vi "Generate Random Lorem Ipsum Error Message.vi"(1 "Dummy Error Message Length":T1=enum."Medium (Up to 1,000 characters)") -> (0 "Random Lorem Ipsum Error Message (dummy error message)":string)   [LabVIEW 2016, in "Simple Tester.lvclass"]
doc: "This VI generates dummy error message. The error messages are based on the Lorem Ipsum text, and are of random lengths."
uses:
  Simple Tester.lvclass
  Dummy Error Message Length (enum).ctl
panel:
  out "Dummy Error Message Length":i32
  out "End index":u32
  out "Input Lorem Ipsum text length":u32
  out "Start index (confirmed)":u32
  out "Start index (randomly chosen)":u32
  # "Development\nControls or indicators that are useful for development or testing, but which are not outputs of the VI."
  # "Input\nInputs to the VI"
  # "Output\nOutputs of the VI"
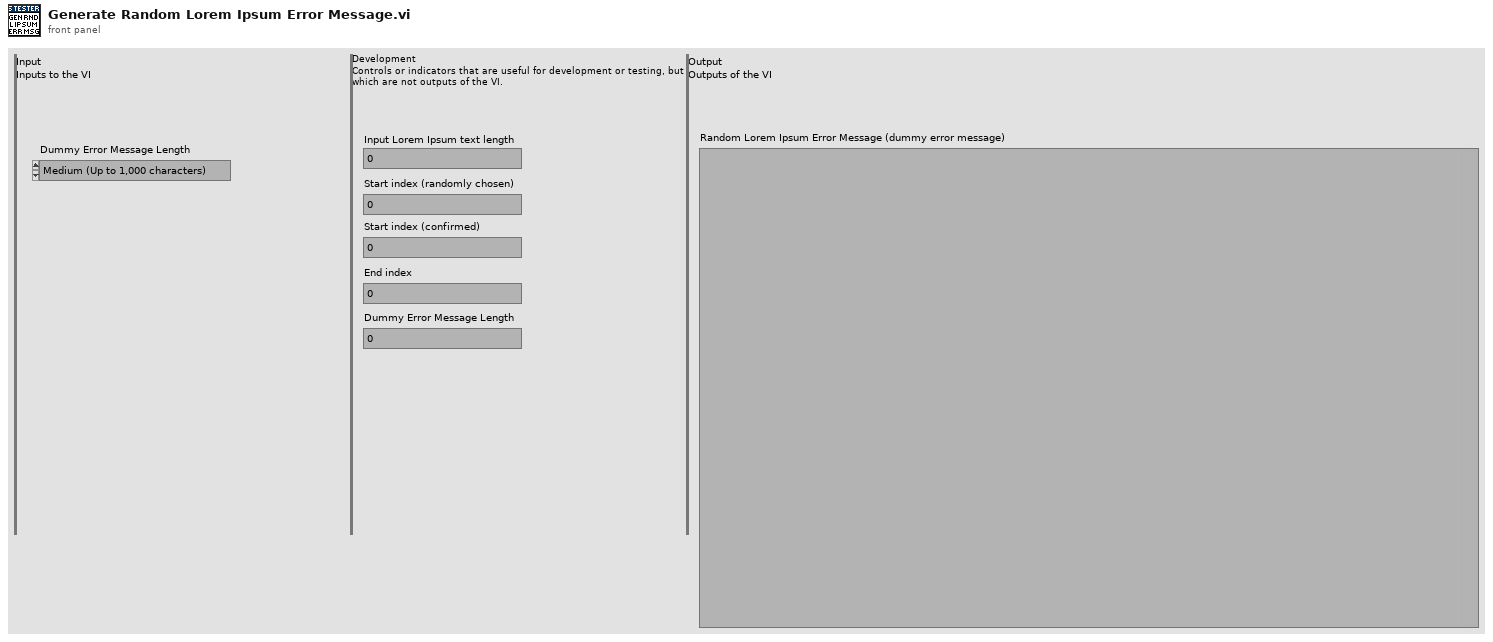
[diagram p1: front panel]
types:
  T1 = typedef "Simple Tester.lvclass/Dummy Error Message Length (enum).ctl" = enum16{"Short (Up to 100 characters)", "Medium (Up to 1,000 characters)", "Long (Up to 10,000 characters)"}
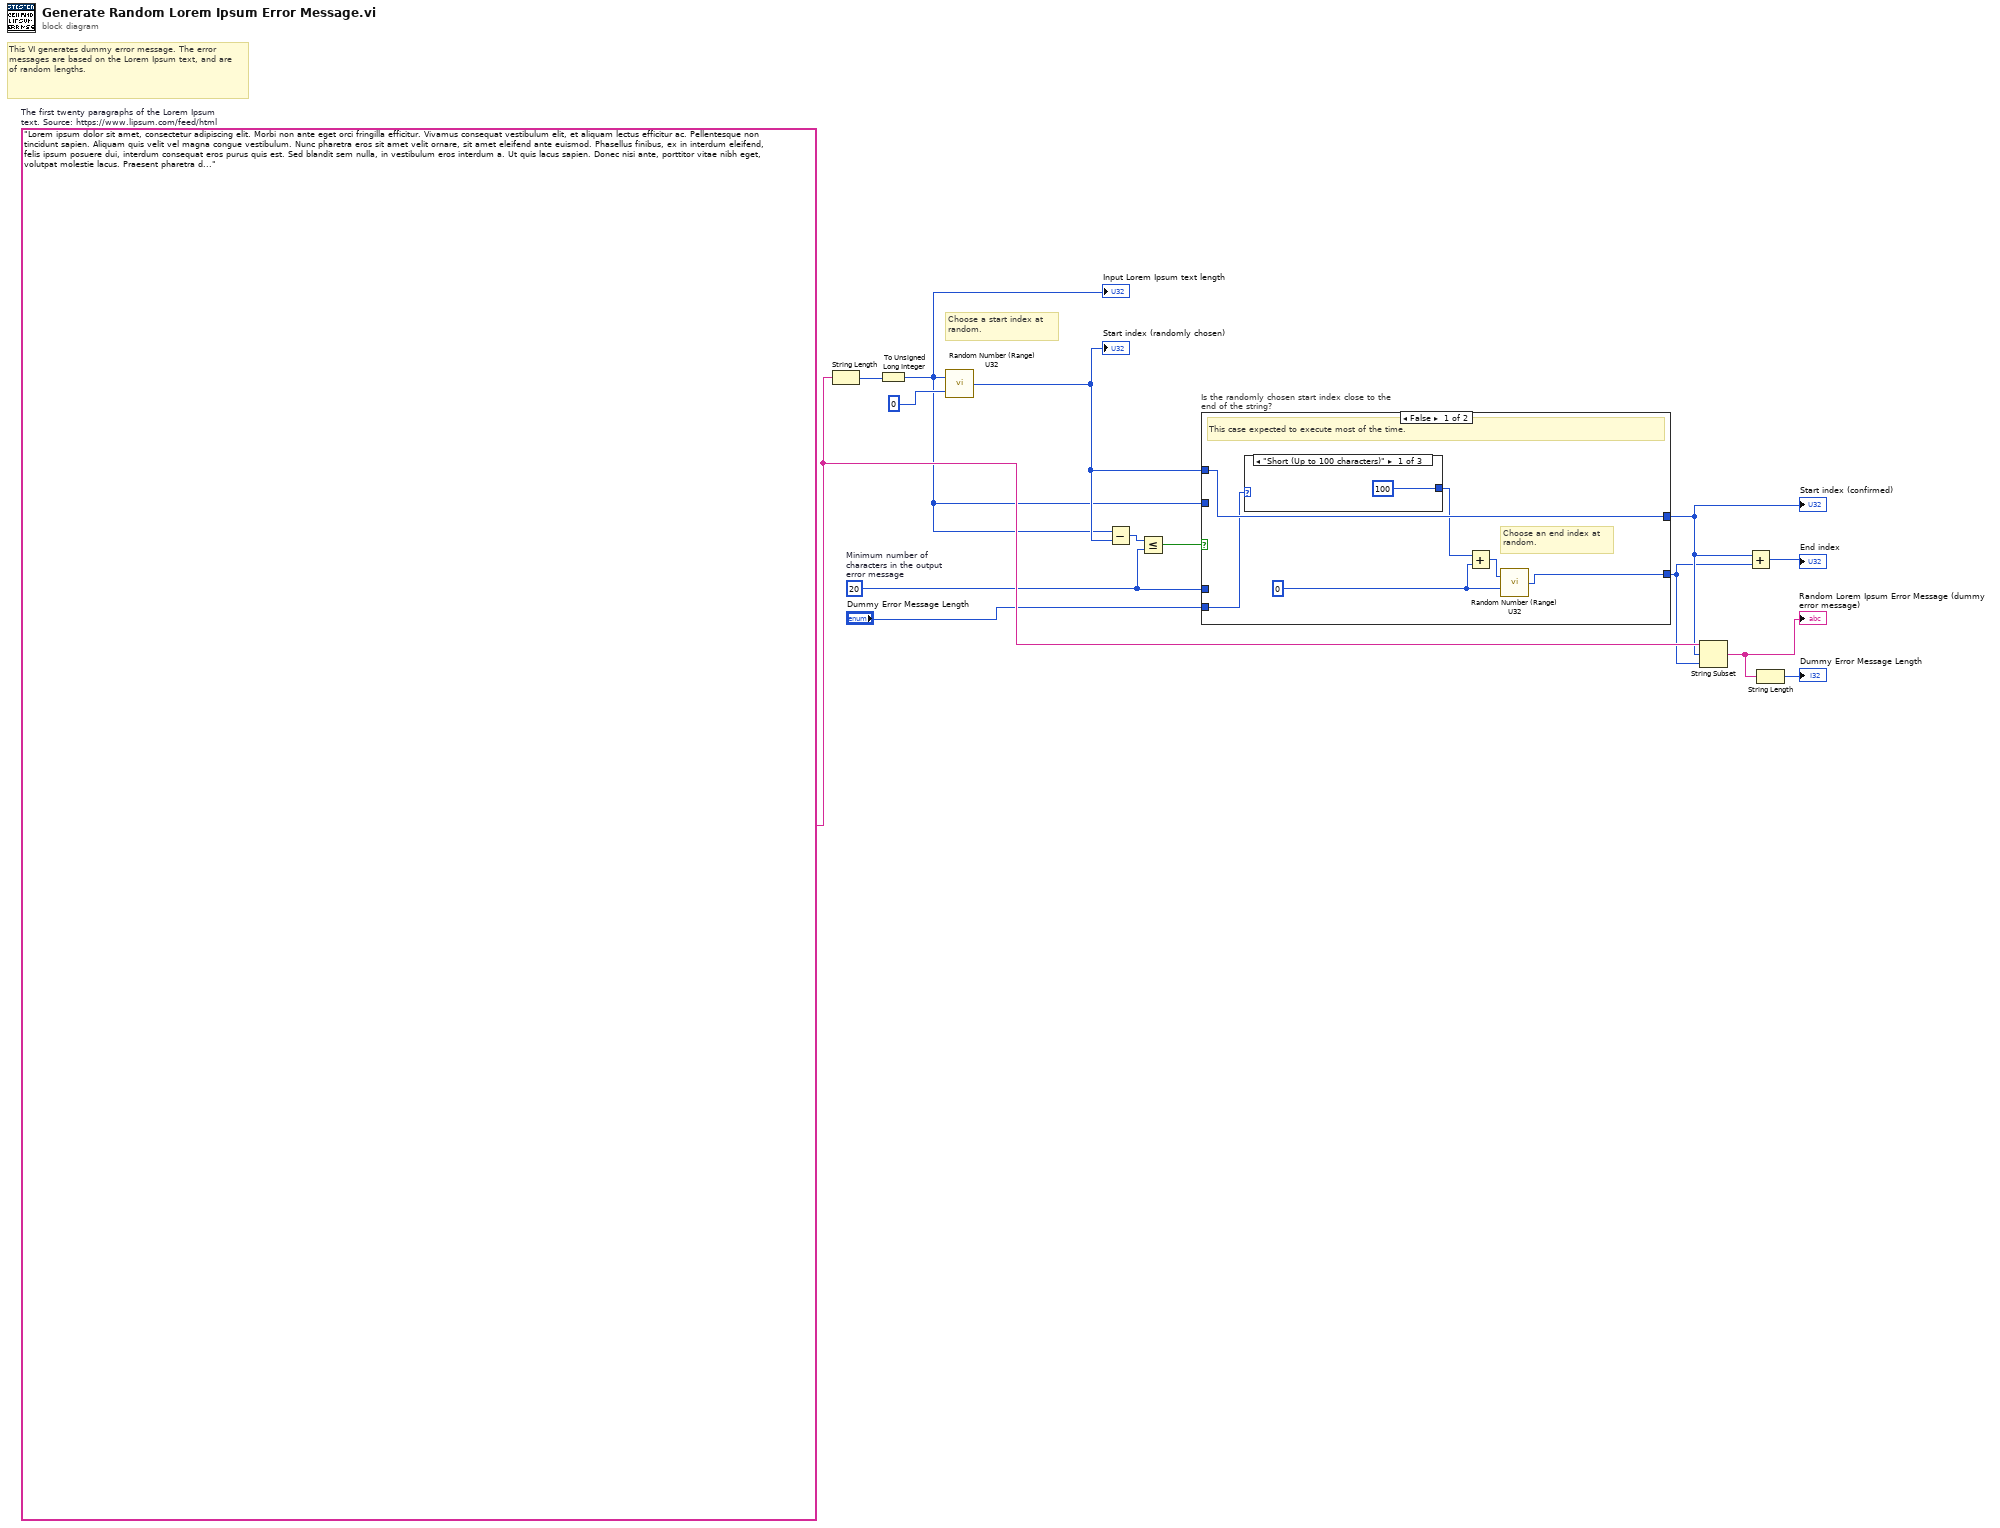
[diagram p0: block diagram]
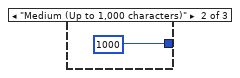
[diagram p2: hidden frame]
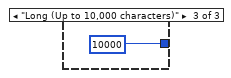
[diagram p3: hidden frame]
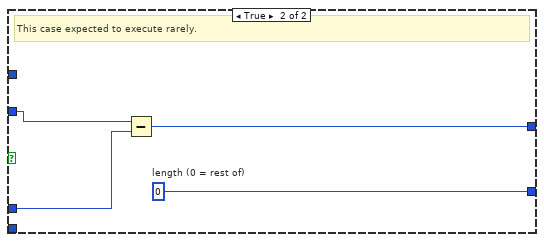
[diagram p4: hidden frame]
diagram:
  w10 = u32 20  # Minimum number of characters in the output error message
  w13 = "Lorem ipsum dolor sit amet, consectetur adipiscing elit. Morbi non ante eget orci fringilla efficitur. Vivamus consequat vestibulum elit, et aliquam lectus efficitur ac. Pellentesque non tincidunt sapien. Aliquam quis velit vel magna congue vestibulum. Nunc pharetra eros sit amet velit ornare, sit amet eleifend ante euismod. Phasellus finibus, ex in interdum eleifend, felis ipsum posuere dui, interdum consequat eros purus quis est. Sed blandit sem nulla, in vestibulum eros interdum a. Ut quis lacus sapien. Donec nisi ante, porttitor vitae nibh eget, volutpat molestie lacus. Praesent pharetra diam vitae dolor cursus, sed finibus tellus convallis. Nullam et sodales dui. Aliquam vehicula pellentesque odio, sed mattis leo gravida consectetur. Aliquam fermentum ex lacus, eget venenatis erat tincidunt vitae. Cras pharetra lacinia elit nec pulvinar.\n\nIn hac habitasse platea dictumst. Donec sit amet quam non justo pharetra lobortis id in justo. Suspendisse aliquet lectus venenatis aliquet scelerisque. Sed imperdiet dictum enim, nec maximus dui pretium condimentum. Aenean vel facilisis eros, et vestibulum mauris. Donec eget libero aliquet, suscipit augue eu, dapibus sapien. Phasellus nunc dui, suscipit sed dui vitae, sollicitudin lacinia turpis.\n\nMaecenas sit amet augue at orci aliquet accumsan a ut mi. Suspendisse ultrices tellus quis nibh pretium luctus. Curabitur sapien orci, pharetra at ligula sit amet, dapibus pulvinar augue. Nullam risus risus, sollicitudin in molestie sed, suscipit ut arcu. Suspendisse non suscipit quam. Quisque fringilla id ante a vehicula. Donec vel maximus ante. Vivamus ut hendrerit lectus. Nunc tincidunt vel nibh id tristique. Pellentesque aliquet libero rutrum tortor vulputate, quis euismod turpis blandit. Phasellus efficitur feugiat convallis. Aliquam lectus ipsum, sodales et velit vel, iaculis mollis est. Nulla quis varius elit. Duis massa elit, feugiat non massa non, interdum dignissim urna. Nunc at velit quis nisl mollis blandit nec sit amet nisi. Sed dignissim ex eu tincidunt ultricies.\n\nUt commodo tempus elit, ac tincidunt dui vehicula et. Suspendisse convallis ante sit amet felis semper ultrices. Donec ultricies bibendum lacus nec laoreet. Etiam ullamcorper felis tellus, in mattis felis pulvinar molestie. Aenean et velit a lacus gravida scelerisque nec ac odio. Aliquam erat volutpat. Nulla facilisi. Maecenas id augue mauris. Ut tempus leo et lectus ultrices elementum. Duis posuere, nisl eget elementum sagittis, justo leo mattis tellus, id aliquam ipsum leo in dui. Praesent ut nisi non ante lobortis gravida. Donec id sem orci.\n\nNam sed lectus sed orci maximus volutpat id et nisi. Vestibulum vulputate consectetur velit et dictum. Sed sit amet ex lacus. Orci varius natoque penatibus et magnis dis parturient montes, nascetur ridiculus mus. Donec consequat lorem sit amet tellus aliquam, at vehicula velit viverra. Sed ipsum turpis, volutpat ac justo eu, suscipit pharetra eros. Duis bibendum auctor orci sit amet eleifend. Vivamus turpis neque, fringilla vitae mattis ac, consequat vel turpis. Donec dapibus sapien eu mauris viverra, a interdum augue lobortis. Nullam vitae ultrices ex. Nulla in purus porttitor elit fringilla sagittis.\n\nQuisque fermentum massa quis lectus finibus faucibus. Nulla aliquet ac arcu in sagittis. Suspendisse nec massa ullamcorper, porta nulla quis, rhoncus enim. Sed ornare rhoncus nulla, sed fringilla ex tincidunt eget. Sed varius ipsum ligula, eu sollicitudin eros lobortis ut. Maecenas tristique nulla erat, sed faucibus erat rhoncus a. Nam elementum nisl quis est cursus, ac tempor mauris feugiat.\n\nDonec vitae maximus justo. Morbi sapien lorem, elementum at pellentesque sed, luctus eu quam. Ut congue efficitur eros id egestas. In ac nunc sed elit ultricies pellentesque. Donec et velit ac ante efficitur malesuada vel sed mi. Donec convallis, mi lacinia convallis tristique, nunc dolor elementum sapien, ac mollis magna sapien a felis. Vivamus at purus pellentesque mauris eleifend tincidunt ut at augue. Suspendisse tristique erat nec neque tristique finibus vel quis nunc. Cras posuere eros mauris, sed ultrices arcu auctor interdum. Quisque ac elit commodo, tempor urna eget, viverra ante. Vestibulum auctor elit sit amet leo blandit, mattis tempus tellus auctor. Donec mollis sem et urna aliquam, at consectetur mi bibendum. Vivamus pellentesque, ex id ullamcorper molestie, justo mauris hendrerit nunc, vitae pretium elit mi ac diam. Praesent efficitur ligula vitae ex ultrices, eget pulvinar purus posuere.\n\nSed efficitur mollis odio, vel semper lorem tempor id. Maecenas blandit arcu eu ante malesuada finibus. Curabitur ut nunc consequat, laoreet risus ac, rhoncus enim. Cras diam neque, consectetur vel faucibus et, pulvinar sed quam. Nam quis feugiat est, eu viverra velit. Maecenas consequat tortor urna, ut facilisis lectus ultrices et. Pellentesque dictum leo id ex tincidunt, sit amet bibendum arcu pretium. Cras maximus facilisis ornare. Integer efficitur augue quis magna tristique, sed scelerisque urna placerat. Etiam ornare neque lectus, eget gravida orci vestibulum nec.\n\nSuspendisse hendrerit congue lorem vel consectetur. Vivamus purus nulla, condimentum vel auctor ut, dignissim vel mi. Lorem ipsum dolor sit amet, consectetur adipiscing elit. Curabitur non gravida ex. Morbi sodales sem id justo eleifend pretium. Duis aliquam mi ut leo ornare porta. Phasellus vehicula tortor mi, a hendrerit elit ultrices vitae. Curabitur nec rutrum orci, non venenatis leo. Maecenas hendrerit orci eu tincidunt efficitur. Integer fringilla finibus iaculis.\n\nNulla facilisi. Proin id mi nec lectus varius aliquam. Nulla porta, velit in varius volutpat, libero massa interdum metus, sit amet mattis est lorem nec felis. Vestibulum ante ipsum primis in faucibus orci luctus et ultrices posuere cubilia curae; Integer aliquam malesuada justo, quis porta quam ultrices in. Nam nec interdum lorem. Praesent metus enim, eleifend a neque nec, aliquet imperdiet erat.\n\nPhasellus tortor justo, tincidunt vitae tempor nec, aliquam nec ipsum. Nulla gravida tortor vel metus efficitur, ut rutrum libero vestibulum. Suspendisse rutrum auctor massa rutrum ullamcorper. In hac habitasse platea dictumst. Integer feugiat vel dui et maximus. Morbi eu mauris eget lectus efficitur vestibulum nec quis libero. Etiam at lectus pellentesque, maximus nisl a, tristique odio. Vivamus pretium libero id justo vestibulum imperdiet.\n\nNulla eu tellus pharetra, egestas nibh ut, vehicula quam. Duis vitae odio non risus hendrerit viverra eget eget enim. Nam eleifend, felis eget vehicula varius, enim nunc facilisis neque, vitae tincidunt eros tortor eget erat. Sed ultrices sapien nibh, vitae maximus ex rutrum sit amet. Nullam in ipsum ut velit maximus mollis nec ultricies urna. Duis et egestas orci. Quisque non magna tortor. In imperdiet tortor diam, eget commodo nunc varius et. In hendrerit imperdiet tellus vitae mollis.\n\nUt euismod nulla id augue elementum, non tempor nibh vulputate. Mauris vulputate ut massa quis vulputate. Nullam tristique elit nisl, sed dignissim mi sollicitudin eu. Vivamus cursus neque mauris, vitae feugiat augue aliquam sit amet. Cras efficitur, nunc vitae tincidunt iaculis, ante orci fermentum leo, vel hendrerit leo est fermentum ligula. Nullam sed erat vitae justo dapibus mattis. Phasellus rutrum scelerisque risus. Nunc auctor sed arcu non venenatis. Ut lectus tellus, semper sit amet nunc vel, dapibus bibendum nunc. Sed interdum, nunc eget rhoncus lacinia, nunc orci ornare nibh, porttitor faucibus arcu elit ut sapien. Suspendisse potenti. Duis ligula augue, facilisis id tellus sed, malesuada tristique erat. Nam fermentum lorem diam, vitae bibendum mauris condimentum nec.\n\nNulla at velit massa. Etiam eu justo ut dui pretium sodales. Aliquam in justo ex. Integer lacinia nunc ut eros porta, quis venenatis felis mattis. Pellentesque elementum nunc lobortis, dictum sem non, bibendum ante. Nulla efficitur ultrices sapien, nec lacinia orci malesuada id. Nullam maximus arcu felis, ac rhoncus quam euismod a. Nam luctus, diam non pulvinar viverra, massa ante mollis massa, ac venenatis lorem odio nec nisi. Nam molestie gravida risus, eu pellentesque erat tincidunt laoreet. Orci varius natoque penatibus et magnis dis parturient montes, nascetur ridiculus mus. Maecenas consequat vestibulum nisl, et malesuada felis commodo ut. Aliquam tincidunt, tellus in egestas dignissim, eros elit sodales metus, vel porttitor odio orci id tortor. Nulla congue condimentum eleifend. Duis a purus elit. In pretium, nisl sit amet volutpat sagittis, mi orci malesuada odio, eget placerat enim purus in lorem. Maecenas molestie velit et lacus posuere, ac mattis massa posuere.\n\nPhasellus dignissim erat in mi semper vehicula. Sed mauris dolor, venenatis ut ullamcorper et, tempor at diam. In euismod vestibulum magna ut sodales. Sed imperdiet condimentum semper. Nunc vel erat at orci posuere semper. Cras sapien purus, auctor quis auctor id, ultrices ac magna. Etiam gravida nec urna eget maximus. Nulla convallis vestibulum nisi, a elementum tortor placerat ac. Nulla ornare aliquet vehicula. Cras ac est a quam pharetra venenatis in ut leo.\n\nNullam ac augue fermentum, commodo justo ac, molestie leo. Integer vitae sollicitudin leo, vel vehicula nisi. Morbi id nulla eu nulla scelerisque euismod. Cras posuere tellus ac risus consequat molestie. Vestibulum et rutrum ante. Quisque pharetra est a consequat ultrices. Maecenas ac molestie neque. Aenean facilisis mauris nec felis laoreet auctor. Vestibulum posuere finibus pellentesque. Mauris ultricies nec libero ac placerat. Ut congue arcu et tincidunt lacinia. Vestibulum sem mi, venenatis id erat ut, mattis fermentum neque.\n\nNunc ante ipsum, viverra eget tincidunt quis, elementum mollis eros. Sed euismod vehicula orci vitae lobortis. Curabitur aliquet, urna quis suscipit blandit, nibh mi malesuada dolor, pharetra feugiat augue lacus eget urna. Nam neque felis, tristique et sapien vel, sollicitudin posuere lectus. Vivamus eget finibus nunc, eu hendrerit mauris. Phasellus pulvinar turpis non auctor hendrerit. Fusce et mi tincidunt, aliquam nulla sit amet, ullamcorper metus. Nunc eget sem eu leo semper dictum. In consequat vestibulum velit interdum laoreet. Etiam interdum neque accumsan varius consequat. Nullam interdum, mi non tristique dictum, metus erat blandit tortor, at dignissim mi ligula et enim.\n\nProin ornare rutrum orci id bibendum. Sed consequat pharetra massa nec faucibus. Vestibulum id odio vel diam sagittis posuere. Nulla vitae tellus massa. Sed mollis consectetur mi id efficitur. Interdum et malesuada fames ac ante ipsum primis in faucibus. Morbi libero felis, pulvinar vitae turpis vel, luctus laoreet eros. Fusce sed ex at leo dignissim tempor ac eget diam. Duis consectetur, urna sed vestibulum mollis, nunc lectus suscipit eros, at ornare lacus velit at felis. In hac habitasse platea dictumst. Curabitur maximus dapibus ligula non vulputate. Nulla sit amet magna sit amet ante pretium interdum a feugiat diam. Cras in sem eu erat dapibus rutrum quis id mi. Etiam ut tristique nibh. Curabitur in lacus velit.\n\nUt vitae massa lacus. Nulla eget est non risus pellentesque rhoncus. Nam posuere orci et est euismod, non varius leo mollis. Pellentesque habitant morbi tristique senectus et netus et malesuada fames ac turpis egestas. Pellentesque gravida mollis leo. Vivamus tempus, orci efficitur scelerisque ultricies, leo nisi tincidunt ipsum, vel condimentum metus odio quis mi. Mauris vitae neque libero. Mauris gravida, augue eget commodo venenatis, justo diam mattis mauris, eu porta odio augue id neque. Donec maximus augue id pellentesque consequat. In hac habitasse platea dictumst. Nam imperdiet quam nibh, vel ornare dui mollis sit amet. Fusce placerat, urna non tincidunt sagittis, nisl nunc dictum sapien, et ultricies magna nulla non nunc.\n\nMorbi diam quam, aliquet non finibus ac, mattis eu massa. Donec aliquet molestie tellus, eu luctus odio lobortis et. Morbi vitae arcu tincidunt, eleifend neque et, semper ante. Aenean viverra ultrices velit, in molestie quam accumsan id. Sed vestibulum neque magna. Morbi aliquam nibh non mauris volutpat pretium. Curabitur lacinia erat erat, vel pulvinar dolor volutpat ut. Sed ornare pulvinar hendrerit. Proin vel fringilla lectus, eget consequat magna. Pellentesque at dolor ut tortor molestie ultrices. Duis sed lectus neque. In ac ante at magna gravida commodo. Aenean ultrices risus vitae tristique tempus."  # The first twenty paragraphs of the Lorem Ipsum text. Source: https://www.lipsum.com/feed/html
  # "Choose a start index at random."
  # "This VI generates dummy error message. The error messages are based on the Lorem Ipsum text, and are of random lengths."
  n1 = String Length(string=w13) -> (length=w5:i32)
  n2 = To Unsigned Long Integer(number=w5) -> (unsigned 32bit integer=w4:u32)
  "Input Lorem Ipsum text length" <- w4
  n3 = call "Random Number (Range) U32.vi"("lower bound"=u32 0 ("lower bound (0)"), "upper bound"=w4) -> ("number"=w9:u32)
  "Start index (randomly chosen)" <- w9
  n4 = Subtract(x=w4, y=w9) -> (x-y=w12:u32)
  n5 = Less Or Equal?(x=w12, y=w10) -> (x <= y?=w11:bool)
  n6 = case "Is the randomly chosen start index close to the end of the string?" shown="False" w11 {
    tunnel: [w19 w27] -> w1
    tunnel: w4 -> [_ w26]
    tunnel: w10 -> [_ w25]
    tunnel: [w20 w24] -> w2
    tunnel: w9 -> [w20 _]
    tunnel: "Dummy Error Message Length" -> [w17 _]
    frame False {
      w18 = u32 0 ("lower bound (0)")
      # "Choose an end index at random."
      # "This case expected to execute most of the time."
      n7 = case shown="\"Short (Up to 100 characters)\"" w17 {
        tunnel: [u32 100 ("lower bound (0)") u32 1000 ("lower bound (0)") u32 10000 ("lower bound (0)")] -> w16
        frame "Short (Up to 100 characters)" {
        }
        frame "Medium (Up to 1,000 characters)" {
        }
        frame "Long (Up to 10,000 characters)" {
        }
      }
      n8 = Add(x=w16, y=w18) -> (x+y=w15:u32)
      n9 = call "Random Number (Range) U32.vi"("lower bound"=w18, "upper bound"=w15) -> ("number"=w19:u32)
    }
    frame True {
      w27 = u32 0  # length (0 = rest of)
      # "This case expected to execute rarely."
      n10 = Subtract(x=w26, y=w25) -> (x-y=w24:u32)
    }
  }
  "Start index (confirmed)" <- w2
  n11 = String Subset(string=w13, offset (0)=w2, length (rest)=w1) -> (substring=w7:string)
  "Random Lorem Ipsum Error Message (dummy error message)" <- w7
  n12 = Add(x=w2, y=w1) -> (x+y=→"End index":u32)
  n13 = String Length(string=w7) -> (length=→"Dummy Error Message Length":i32)
